vi "RealSense_HelloWorld_PointCloud_ext_RGB2.vi"() -> ()   [LabVIEW 2017]
doc: "Simple Demo showing how to connect a RealSense Camera to stream COLOR and DEPTH from the stereo camera of a D4xx series camera."
uses:
  libRealSense3.lvlib
  <vilib>/picture/3D Picture Control/NI_3D Picture Control.lvlib
  <vilib>/Utility/miscctls.llb/LV3DPointTypeDef.ctl
  <vilib>/Utility/miscctls.llb/LVRGBAColorTypeDef.ctl
  <vilib>/picture/3D Picture Control/Object/Create Object (name).vi
panel:
  in  "stop and exit":bool
  in  "Display tab":T1(tab)=enum."Color + Depth"
  out "RGB height":i32=720
  out "RGB width":i32=1280
  in  "Select RGB Resolution":u16(ring)=30 items=["320 x 180 @6fps", "320 x 180 @15fps", "320 x 180 @30fps", "320 x 180 @60fps", "320 x 240 @6fps", "320 x 240 @15fps", "320 x 240 @30fps", "320 x 240 @60fps", "424 x 240 @6fps", "424 x 240 @15fps", "424 x 240 @30fps", "424 x 240 @60fps", "640 x 360 @6fps", "640 x 360 @15fps", "640 x 360 @30fps", "640 x 360 @60fps", "640 x 480 @6fps", "640 x 480 @15fps", "640 x 480 @30fps", "640 x 480 @60fps", "848 x 480 @6fps", "848 x 480 @15fps", "848 x 480 @30fps", "848 x 480 @60fps", "960 x 540 @6fps", "960 x 540 @15fps", "960 x 540 @30fps", "960 x 540 @60fps", "1280 x 720 @6fps", "1280 x 720 @15fps", "1280 x 720 @30fps", "1920 x 1080 @6fps", "1920 x 1080 @15fps", "1920 x 1080 @30fps"]
  out "Depth height":i32=720
  out "Depth width":i32=1280
  out "init results":T2={"camera name"="Intel RealSense D435I", "camera S/N"="834412070342", "F/W"="05.12.01.00", "Sensor name"="Stereo Module", "api_version"=23201, "rscontext"=1659248689968, "device_list"=1659375430384, "device count"=1, "Dev out"=1659375543056, "sensor_list"=1659375327152, "sensor count"=3, "Sensor out"=1659374593968}
  in  "Select Depth Resolution":u16(ring)=32 items=["424 x 240 @6fps", "424 x 240 @15fps", "424 x 240 @30fps", "424 x 240 @60fps", "424 x 240 @90fps", "480 x 270 @6fps", "480 x 270 @15fps", "480 x 270 @30fps", "480 x 270 @60fps", "480 x 270 @90fps", "640 x 360 @6fps", "640 x 360 @15fps", "640 x 360 @30fps", "640 x 360 @60fps", "640 x 360 @90fps", "640 x 480 @6fps", "640 x 480 @15fps", "640 x 480 @30fps", "640 x 480 @60fps", "640 x 480 @90fps", "848 x 100 @6fps", "848 x 100 @15fps", "848 x 100 @30fps", "848 x 100 @60fps", "848 x 100 @90fps", "848 x 480 @6fps", "848 x 480 @15fps", "848 x 480 @30fps", "848 x 480 @60fps", "848 x 480 @90fps", "1280 x 720 @6fps", "1280 x 720 @15fps", "1280 x 720 @30fps", "1280 x 720 @60fps"]
  in  "Sensor index":i32
  in  "Device index":i32
  out "L-R Baseline, mm":sgl=-49.906834
  out "fy":sgl=656.61536 format="%#_5g"
  out "fx":sgl=656.61536 format="%#_5g"
  out "ppy":sgl=357.01468 format="%#_5g"
  out "ppx":sgl=632.28015 format="%#_5g"
  out "RGB Sensor":T3={"Sensor info"="RGB Camera", "Sensor out"=1659374594288, "error"=0}
  out "Stream Profile Handles":u64[](array[numeric])=[1659375449352]
  out "queue out":u64=1659245873280
  out "sensor out":u64=1659374594288
  out "Sensor out":u64=1659374594288
  out "Stream type":u16(ring)=2 items=["Depth"=0, "Color (ext.)"=2, "Color (left) "=3, "IR Left"=5, "IR Right"=9, "IR Left (Y16)"=21, "IR Right (Y16)"=25]
  in  "Exposure,us":sgl=33000.0
  in  "Autoexposure":bool=TRUE
  in  "Depth Presets":T4(ring)=enum."Face2"
  in  "Color Presets":T5(ring)=enum."DS410 (DS5a) 4"
  in  "Laser on/off":bool=TRUE
  in  "Gain(16-248)":sgl=16.0 min=16 max=248
  in  "Update Presets":bool
  in  "Laser \nPower (mW)":dbl(slide)=155.72448 min=0.0 max=360.0 scale=0.36..360.0
  in  "Range Scale":enum16{"200m", "100m", "60m", "6m", "2m", "1m"}(ring)=enum."6m"
  out "RGB image":picture
  out "Depth map":sgl[][](graph)
  out "3D Picture":refnum<vi>(3d-picture)
  out "RGB capture error":string="No Error"
  out "init error":string="\rNo Error\rNo Error\rNo Error\rNo Error\rNo Error\rNo Error\rNo Error\r\rNo Error\rNo Error"
  out "Depth Capture":string="No Error"
  out "Start Error":string="No Error\rNo Error\rNo Error"
  out "Config error":string="No Error\rNo Error"
  out "Close Error":string="No Error\rNo Error\rNo Error\rNo Error"
  out "release frame error":string="No Error"
  out "iteration":i32=762
  in  "stop":bool=TRUE
  # "RealSense Hello World: PointCloud ext. RGB"
  # "This demo shows how to connect a RealSense D435(e) & D415(e) Stereo Depth Camera, and display the textured PointCloud."
  # "Note; When you change Depth Preset you need to stop and restart for the HDAD settings to take effect.\n\nTry the Color preset called \"Remove IR2\". It will remove the laser projector from the RGB 1280x720 image."
  # "INTRINSICS & EXTRINSICS"
  # "SELECT THE RESOLUTION"
  # "DEPTH MAP"
  # "COLOR"
  # "Changes Color scale for Depth Map."
  # "20-1660000"
  # "3D POINTCLOUD"
  # "Rotate: Drag image\nMove X-Y: HOLD DOWN CTRL while dragging.\nZoom: SHIFT while dragging."
  # "ERRORS"
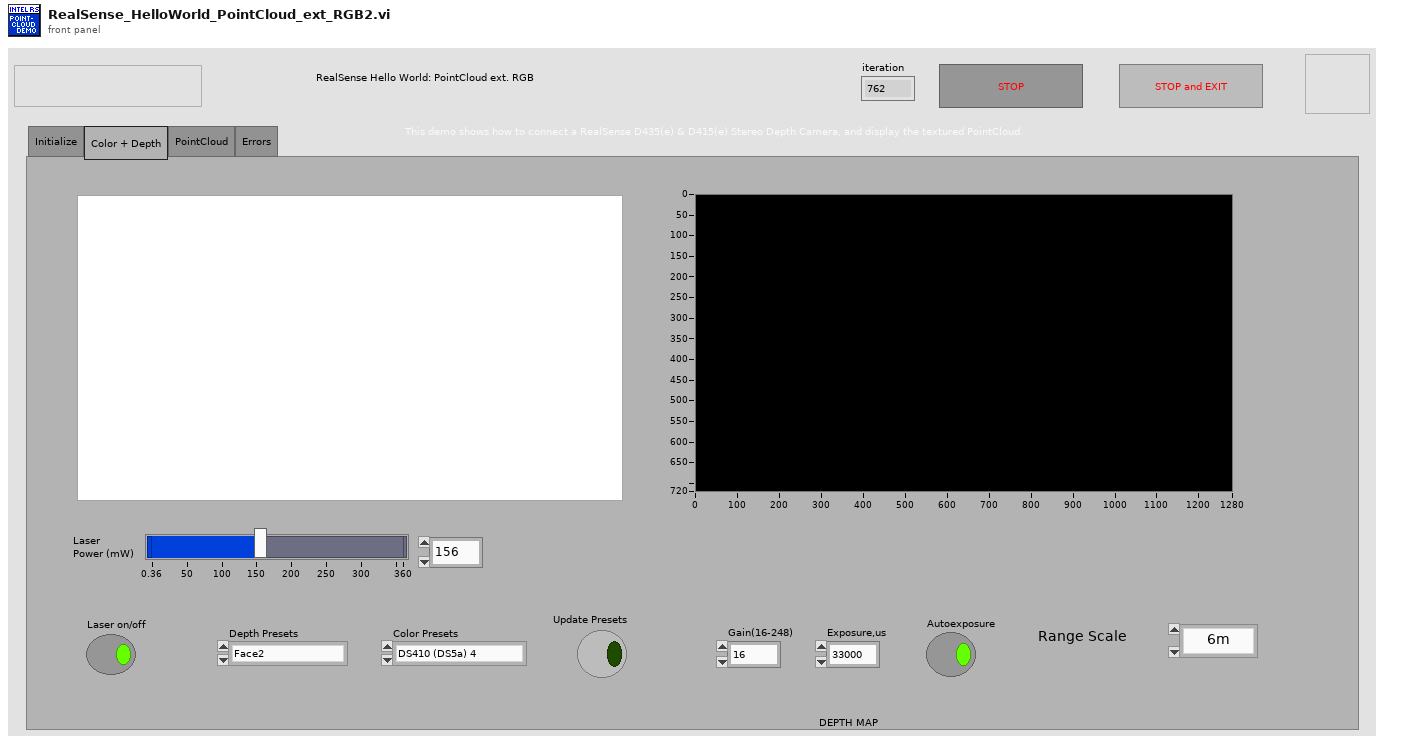
[diagram p1: front panel]
types:
  T1 = enum32{"Initialize", "Color + Depth", "PointCloud", "Errors"}
  T2 = cluster{"camera name":string, "camera S/N":string, "F/W":string, "Sensor name":string, "api_version":i32, "rscontext":u64, "device_list":u64, "device count":i32, "Dev out":u64, "sensor_list":u64, "sensor count":i32, "Sensor out":u64}
  T3 = cluster{"Sensor info":string, "Sensor out":u64, "error":u64}
  T4 = enum16{"Custom", "Original", "New Depth 1", "New Depth 2", "Depth Active 1", "Active 3D Scan", "Active Short A", "Active Short C", "Face", "Face2", "Best Box", "High Density", "Medium Density", "High Accuracy", "Hand", "Short Range", "Flat wall", "Load .JSON", "Load .JSON2"}
  T5 = enum16{"Custom", "RS400 (DS5p)", "RS400 (DS5p) 2", "RS400 (DS5p) 3", "RS400 (DS5p) 4", "RS400 (DS5p) 5", "RS410 (DS5a)", "RS410 (DS5a) 2", "DS410 (DS5a) 3", "DS410 (DS5a) 4", "DS410+IR", "DS5LR", "DS5LR-2", "DS5LR no pattern", "RS410 Remove IR", "RS410 Remove IR 2", "DS5micro", "D435"}
  T6 = cluster{"Sensor info":string, "Sensor out":u64, "error":u64}[]
  T7 = cluster{"width":i32, "height":i32, "fps":i32, "Profile":u64, "ppx":sgl, "ppy":sgl, "fx":sgl, "fy":sgl, "model":u32}
  T8 = enum16{"Overall", "Per Primitive", "Per Vertex", "Binding Off"}
  T9 = enum16{"Points", "Lines", "Line Strip", "Line Loop", "Triangles", "Triangle Strip", "Triangle Fan", "Quads", "Quad Strip", "Polygon"}
  T10 = cluster{"R":dbl, "G":dbl, "B":dbl, "Alpha":dbl}[]
  T11 = typedef "LVRGBAColorTypeDef.ctl" = cluster{"Red":sgl, "Green":sgl, "Blue":sgl, "Alpha":sgl}
  T12 = typedef "LV3DPointTypeDef.ctl" = cluster{"X":sgl, "Y":sgl, "Z":sgl}
  T13 = cluster{"Alpha":sgl, "Blue":sgl, "Green":sgl, "Red":sgl}
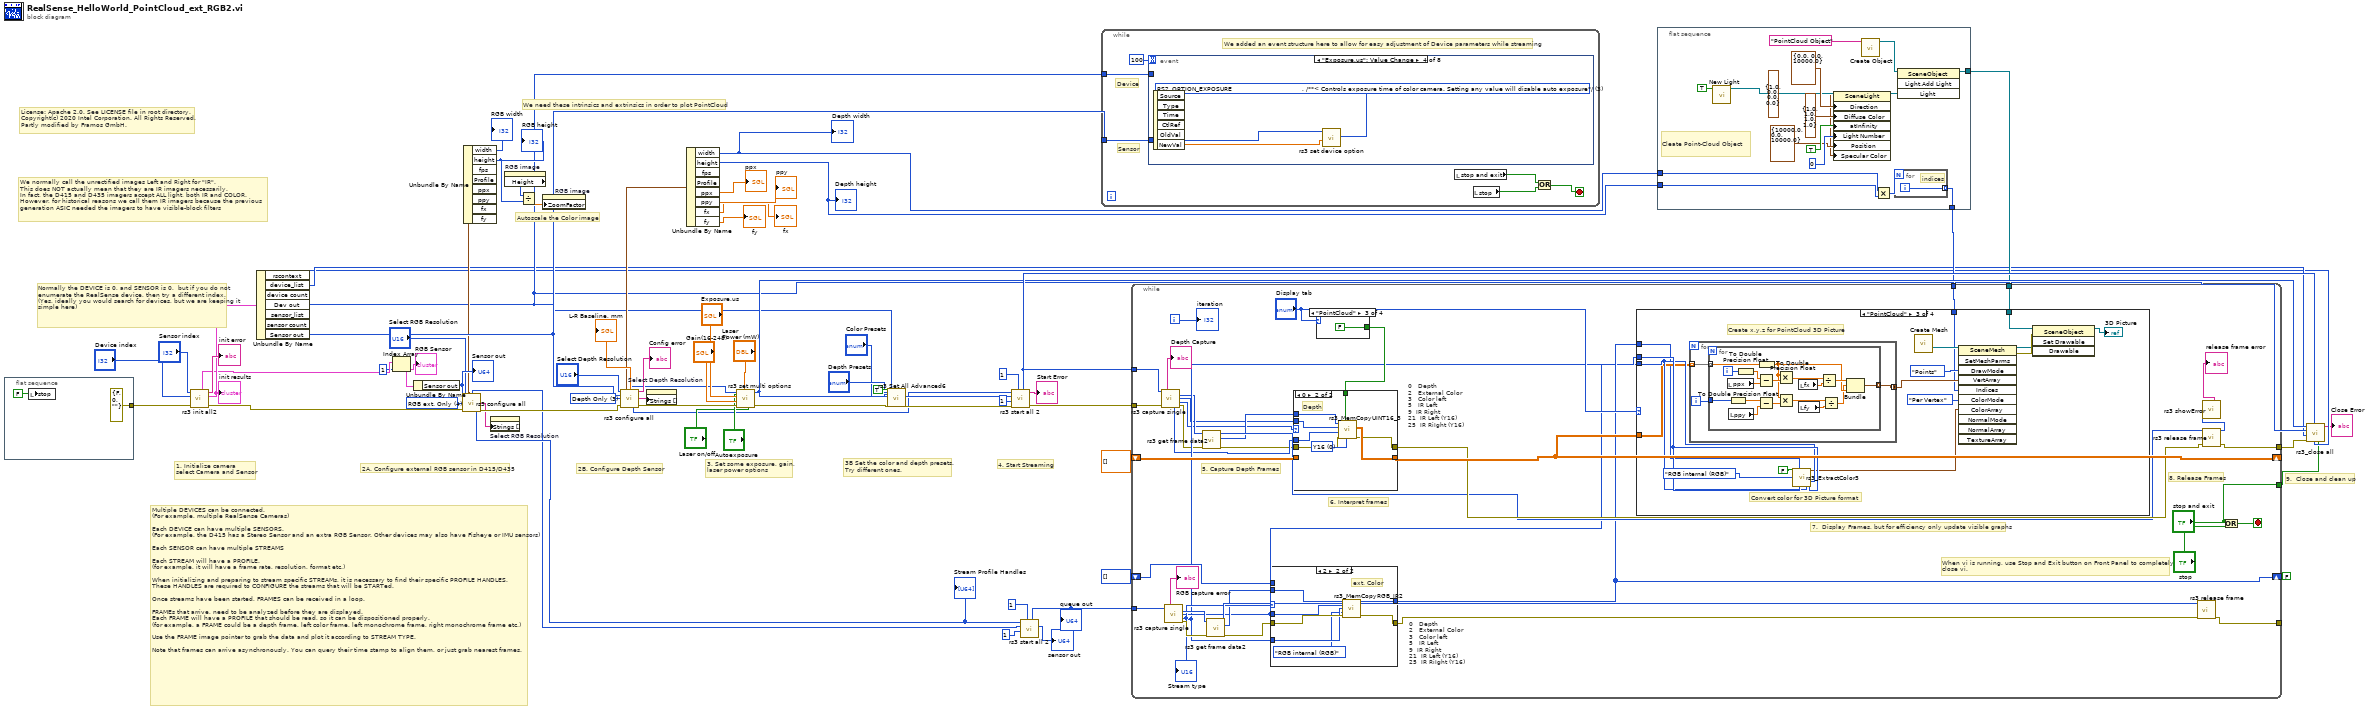
[diagram p0: block diagram]
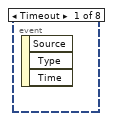
[diagram p2: hidden frame]
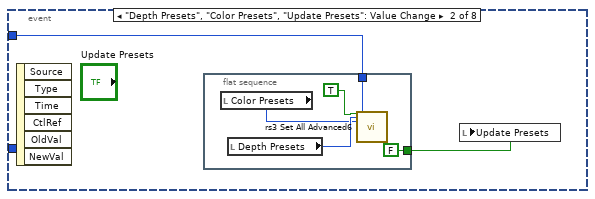
[diagram p3: hidden frame]
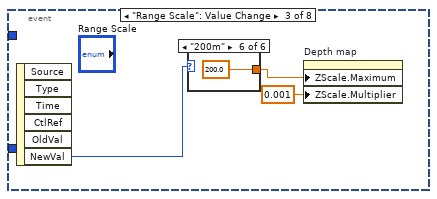
[diagram p4: hidden frame]
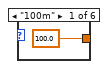
[diagram p5: hidden frame]
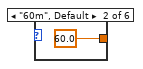
[diagram p6: hidden frame]
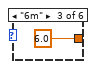
[diagram p7: hidden frame]
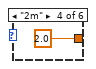
[diagram p8: hidden frame]
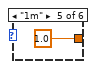
[diagram p9: hidden frame]
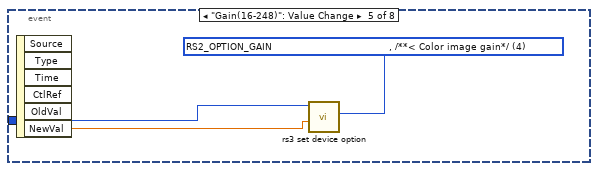
[diagram p10: hidden frame]
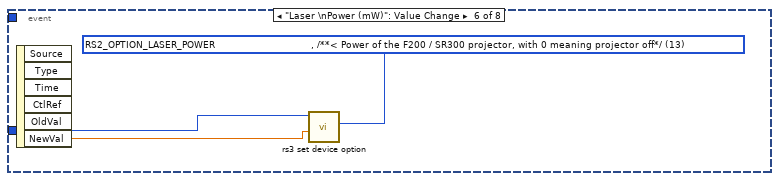
[diagram p11: hidden frame]
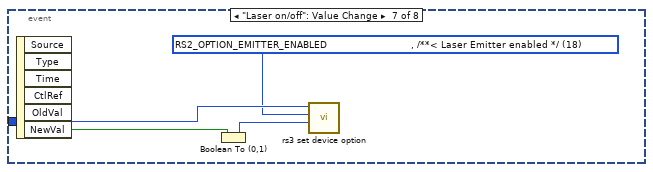
[diagram p12: hidden frame]
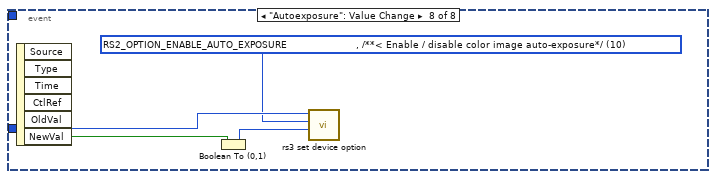
[diagram p13: hidden frame]
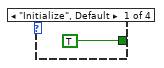
[diagram p16: hidden frame]
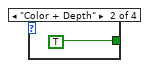
[diagram p17: hidden frame]
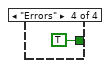
[diagram p18: hidden frame]
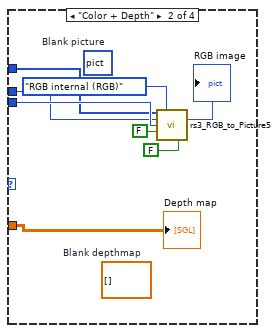
[diagram p20: hidden frame]
diagram:
  (unwired) FALSE
  w21 = u16 4 items=["Depth + Left Color", "Unrectified L + R", "Rectified L + R", "Depth Only", "RGB ext. Only"] ("Stream selection")
  w56 = u16 3 items=["Depth + Left Color", "Unrectified L + R", "Rectified L + R", "Depth Only", "RGB ext. Only"] ("Stream selection")
  # "License: Apache 2.0. See LICENSE file in root directory.\nCopyright(c) 2020 Intel Corporation. All Rights Reserved.\nPartly modified by Framos GmbH."
  # "2A. Configure external RGB sensor in D415/D435"
  # "Autoscale the Color image"
  # "We need these intrinsics and extrinsics in order to plot PointCloud"
  # "3B Set the color and depth presets.\nTry different ones."
  # "We normally call the unrectified images Left and Right for \"IR\". \nThis does NOT actually mean that they are IR imagers necessarily. \nIn fact, the D415 and D435 imagers accept ALL light, both IR and COLOR.\nHowever, for historical reasons we call them IR imagers because the previous generation ASIC needed the imagers to have visible-block filters"
  # "Normally the DEVICE is 0, and SENSOR is 0,  but if you do not enumerate the RealSense device, then try a different index.\n(Yes, ideally you would search for devices, but we are keeping it simple here)"
  # "Multiple DEVICES can be connected. \n(For example, multiple RealSense Cameras)\n\nEach DEVICE can have multiple SENSORS. \n(For example, the D415 has a Stereo Sensor and an extra RGB Sensor. Other devices may also have Fisheye or IMU sensors) \n\nEach SENSOR can have multiple STREAMS\n\nEach STREAM will have a PROFILE. \n(for example, it will have a frame rate, resolution, format etc.)\n\nWhen initializing and preparing to stream specific STREAMs, it is necessary to find their specific PROFILE HANDLES.\nThese HANDLES are required to CONFIGURE the streams that will be STARTed. \n\nOnce streams have been started, FRAMES can be received in a loop. \n \nFRAMEs that arrive, need to be analyzed before they are displayed. \nEach FRAME will have a PROFILE that should be read, so it can be dispositioned properly.\n(for example, a FRAME could be a depth frame, left color frame, left monochrome frame, right monochrome frame etc.)\n\nUse the FRAME image pointer to grab the data and plot it according to STREAM TYPE.\n\nNote that frames can arrive asynchronously. You can query their time stamp to align them, or just grab nearest frames."
  # "9.  Close and clean up"
  # "4. Start Streaming"
  # "3. Set some exposure, gain, \nlaser power options"
  # "2B. Configure Depth Sensor"
  # "1. Initialize camera\nselect Camera and Sensor"
  n1 = flat-sequence {
    tunnel: [errorcluster {"status"=FALSE, "code"=0, "source"=""} ("error in")] -> w57
    frame #0 {
      n2 = local write "stop"(FALSE ("stop")) -> ()
    }
  }
  n3 = call "rs3 init all2.vi"("error in"=w57, "Select Device"="Device index", "Select Sensor"="Sensor index") -> ("error out"=w27:errorcluster, "init results"=w62:T2, "init error"=→"init error":string, "Sensor Array"=w31:T6)  [unwired: 2 in, 3 out]
  "init results" <- w62
  n4 = Unbundle By Name(w62) -> ("rscontext"=w9:u64, "device_list"=w11:u64, "Dev out"=w12:u64, "Sensor out"=w44:u64)  [unwired: 3 out]
  n5 = Index Array(array=w31, index=1) -> (element=w29:T3)
  "RGB Sensor" <- w29
  n6 = Unbundle By Name(w29) -> ("Sensor out"=w28:u64)
  "Sensor out" <- w28
  n7 = call "rs3 configure all.vi"("Select Resolution"="Select RGB Resolution", "Sensor in"=w28, "Stream selection"=w21, "error in (no error)"=w27) -> ("Output stream L"=w24:T7, "Sensor out"=w18:u64, "Output stream"=w8:string[], "Stream Profile Handles"=w19:u64[], "error out"=w25:errorcluster)  [unwired: 2 in, 5 out]
  "Stream Profile Handles" <- w19
  n8 = Unbundle By Name(w24) -> ("width"=→"RGB width":i32, "height"=w22:i32)  [unwired: 6 out]
  "RGB height" <- w22
  n9 = property on="Select RGB Resolution" class="Ring (strict)"("Strings []"=w8) -> ()  [unwired: 2 in, 2 out]
  n10 = property on="RGB image" class="Pict"() -> ("Height"=w40:u32)  [unwired: 2 in, 2 out]
  n11 = Divide(x=w40, y=w22) -> (x/y=w39:dbl)
  n12 = property on="RGB image" class="Pict"("ZoomFactor"=w39) -> ()  [unwired: 2 in, 2 out]
  n13 = call "rs3 configure all.vi"("Select Resolution"="Select Depth Resolution", "Sensor in"=w44, "Stream selection"=w56, "error in (no error)"=w25) -> ("Output stream L"=w41:T7, "Sensor out"=w32:u64, "config error"=→"Config error":string, "Output stream"=w58:string[], "L-R Baseline, mm"=→"L-R Baseline, mm":sgl, "Stream Profile Handles"=w20:u64[], "error out"=w55:errorcluster)  [unwired: 2 in, 3 out]
  n14 = property on="Select Depth Resolution" class="Ring (strict)"("Strings []"=w58) -> ()  [unwired: 2 in, 2 out]
  n15 = Unbundle By Name(w41) -> ("width"=w3:i32, "height"=w2:i32, "ppx"=→"ppx":sgl, "ppy"=→"ppy":sgl, "fx"=→"fx":sgl, "fy"=→"fy":sgl)  [unwired: 2 out]
  "Depth height" <- w2
  "Depth width" <- w3
  n16 = call "rs3 set multi options.vi"("laser on/off"="Laser on/off", "autoexposure"="Autoexposure", "Laser power, mW (0-360)"="Laser \nPower (mW)", "error in (no error)"=w55, "Gain(16-248)"="Gain(16-248)", "Exposure, us"="Exposure,us", "Sensor in"=w32) -> ("error out"=w49:errorcluster, "Sensor out"=w54:u64)  [unwired: 2 in, 1 out]
  n17 = call "rs3 Set All Advanced6.vi"("Set Color Corr"=TRUE, "Depth Presets"="Depth Presets", "Color Presets"="Color Presets", "error in (no error)"=w49, "device in"=w12) -> ("error out"=w48:errorcluster)  [unwired: 20 in, 2 out]
  n18 = call "rs3 start all 2.vi"("capacity"=1, "error in (no error)"=w48, "Count of Streams"=1, "Sensor in"=w54, "Stream profile array"=w20) -> ("error out"=w59:errorcluster, "Config Error"=→"Start Error":string, "queue out"=w65:u64)  [unwired: 3 in, 1 out]
  n19 = call "rs3 start all 2.vi"("capacity"=1, "Count of Streams"=1, "Sensor in"=w18, "Stream profile array"=w19) -> ("sensor out"=→"sensor out":u64, "queue out"=w10:u64)  [unwired: 4 in, 2 out]
  "queue out" <- w10
  n20 = while {
    tunnel: w12 -> [w75]
    tunnel: w44 -> [w74]
    stop <- w70 stop-if-true
    # "Sensor"
    # "Device"
    # "We added an event structure here to allow for easy adjustment of Device parameters while streaming"
    n21 = event shown="[3] \"Exposure,us\": Value Change" {
      selector: _ -> [_ _ _ _ _ _ _ _]
      dyn-events: _ -> [_ _ _ _ _ _ _ _]
      timeout: 100 -> [_ _ _ _ _ _ _ _]
      tunnel: w75 -> [_ w77 _ _ _ _ _ _]
      tunnel: w74 -> [_ _ _ w94 w97 w100 w104 w108]
      event Timeout {
        n22 = event-data() -> ()  [unwired: 1 in, 3 out]
      }
      event "Depth Presets", "Color Presets", "Update Presets": Value Change {
        n23 = event-data() -> ()  [unwired: 1 in, 6 out]
        n24 = flat-sequence {
          tunnel: w77 -> [w79]
          tunnel: [FALSE ("Update Presets")] -> w76
          frame #0 {
            n25 = local read "Color Presets"() -> (w81:T5)
            n26 = local read "Depth Presets"() -> (w82:T4)
            n27 = call "rs3 Set All Advanced6.vi"("Set Color Corr"=TRUE, "Depth Presets"=w82, "Color Presets"=w81, "device in"=w79) -> ()  [unwired: 21 in, 3 out]
          }
        }
        n28 = local write "Update Presets"(w76) -> ()
      }
      event "Range Scale": Value Change {
        n29 = event-data() -> ("NewVal"=w84:enum16{"200m", "100m", "60m", "6m", "2m", "1m"})  [unwired: 1 in, 5 out]
        n30 = case shown="\"200m\"" w84 {
          tunnel: [100.0 ("Z Scale.Offset and Multiplier:Multiplier") 60.0 ("Z Scale.Offset and Multiplier:Multiplier") 6.0 ("Z Scale.Offset and Multiplier:Multiplier") 2.0 ("Z Scale.Offset and Multiplier:Multiplier") 1.0 ("Z Scale.Offset and Multiplier:Multiplier") 200.0 ("Z Scale.Offset and Multiplier:Multiplier")] -> w83
          frame "100m" {
          }
          frame "60m", Default {
          }
          frame "6m" {
          }
          frame "2m" {
          }
          frame "1m" {
          }
          frame "200m" {
          }
        }
        n31 = property on="Depth map" class="IntGraph (strict)"("ZScale.Maximum"=w83, "ZScale.Multiplier"=0.001 ("Z Scale.Offset and Multiplier:Multiplier")) -> ()  [unwired: 2 in, 2 out]
      }
      event "Exposure,us": Value Change {
        w92 = u16 3 items=["    RS2_OPTION_BACKLIGHT_COMPENSATION                     , /**< Enable / disable color backlight compensation*/", "    RS2_OPTION_BRIGHTNESS                                 , /**< Color image brightness*/", "    RS2_OPTION_CONTRAST                                   , /**< Color image contrast*/", "    RS2_OPTION_EXPOSURE                                   , /**< Controls exposure time of color camera. Setting any value will disable auto exposure*/", "    RS2_OPTION_GAIN                                       , /**< Color image gain*/", "    RS2_OPTION_GAMMA                                      , /**< Color image gamma setting*/", "    RS2_OPTION_HUE                                        , /**< Color image hue*/", "    RS2_OPTION_SATURATION                                 , /**< Color image saturation setting*/", "    RS2_OPTION_SHARPNESS                                  , /**< Color image sharpness setting*/", "    RS2_OPTION_WHITE_BALANCE                              , /**< Controls white balance of color image. Setting any value will disable auto white balance*/", "    RS2_OPTION_ENABLE_AUTO_EXPOSURE                       , /**< Enable / disable color image auto-exposure*/", "    RS2_OPTION_ENABLE_AUTO_WHITE_BALANCE                  , /**< Enable / disable color image auto-white-balance*/", "    RS2_OPTION_VISUAL_PRESET                              , /**< Provide access to several recommend sets of option presets for the depth camera */", "    RS2_OPTION_LASER_POWER                                , /**< Power of the F200 / SR300 projector, with 0 meaning projector off*/", "    RS2_OPTION_ACCURACY                                   , /**< Set the number of patterns projected per frame. The higher the accuracy value the more patterns projected. Increasing the number of patterns help to achieve better accuracy. Note that this c", "    RS2_OPTION_MOTION_RANGE                               , /**< Motion vs. Range trade-off, with lower values allowing for better motion sensitivity and higher values allowing for better depth range*/", "    RS2_OPTION_FILTER_OPTION                              , /**< Set the filter to apply to each depth frame. Each one of the filter is optimized per the application requirements*/", "    RS2_OPTION_CONFIDENCE_THRESHOLD                       , /**< The confidence level threshold used by the Depth algorithm pipe to set whether a pixel will get a valid range or will be marked with invalid range*/", "    RS2_OPTION_EMITTER_ENABLED                            , /**< Laser Emitter enabled */", "    RS2_OPTION_FRAMES_QUEUE_SIZE                          , /**< Number of frames the user is allowed to keep per stream. Trying to hold-on to more frames will cause frame-drops.*/", "    RS2_OPTION_TOTAL_FRAME_DROPS                          , /**< Total number of detected frame drops from all streams */", "    RS2_OPTION_AUTO_EXPOSURE_MODE                         , /**< Auto-Exposure modes: Static, Anti-Flicker and Hybrid */", "    RS2_OPTION_POWER_LINE_FREQUENCY                       , /**< Power Line Frequency control for anti-flickering Off/50Hz/60Hz/Auto */", "    RS2_OPTION_ASIC_TEMPERATURE                           , /**< Current Asic Temperature */", "    RS2_OPTION_ERROR_POLLING_ENABLED                      , /**< disable error handling */", "    RS2_OPTION_PROJECTOR_TEMPERATURE                      , /**< Current Projector Temperature */", "    RS2_OPTION_OUTPUT_TRIGGER_ENABLED                     , /**< Enable / disable trigger to be outputed from the camera to any external device on every depth frame */", "    RS2_OPTION_MOTION_MODULE_TEMPERATURE                  , /**< Current Motion-Module Temperature */", "    RS2_OPTION_DEPTH_UNITS                                , /**< Number of meters represented by a single depth unit */", "    RS2_OPTION_ENABLE_MOTION_CORRECTION                   , /**< Enable/Disable automatic correction of the motion data */", "    RS2_OPTION_AUTO_EXPOSURE_PRIORITY                     , /**< Allows sensor to dynamically ajust the frame rate depending on lighting conditions */", "    RS2_OPTION_COUNT                                      , /**< Number of enumeration values. Not a valid input: intended to be used in for-loops. */"] ("RS Option")
        n32 = event-data() -> ("NewVal"=w93:sgl)  [unwired: 1 in, 5 out]
        n33 = call "rs3 set device option.vi"("value"=w93, "RS Option"=w92, "Sensor in"=w94) -> ()  [unwired: 6 in, 3 out]
      }
      event "Gain(16-248)": Value Change {
        w95 = u16 4 items=["    RS2_OPTION_BACKLIGHT_COMPENSATION                     , /**< Enable / disable color backlight compensation*/", "    RS2_OPTION_BRIGHTNESS                                 , /**< Color image brightness*/", "    RS2_OPTION_CONTRAST                                   , /**< Color image contrast*/", "    RS2_OPTION_EXPOSURE                                   , /**< Controls exposure time of color camera. Setting any value will disable auto exposure*/", "    RS2_OPTION_GAIN                                       , /**< Color image gain*/", "    RS2_OPTION_GAMMA                                      , /**< Color image gamma setting*/", "    RS2_OPTION_HUE                                        , /**< Color image hue*/", "    RS2_OPTION_SATURATION                                 , /**< Color image saturation setting*/", "    RS2_OPTION_SHARPNESS                                  , /**< Color image sharpness setting*/", "    RS2_OPTION_WHITE_BALANCE                              , /**< Controls white balance of color image. Setting any value will disable auto white balance*/", "    RS2_OPTION_ENABLE_AUTO_EXPOSURE                       , /**< Enable / disable color image auto-exposure*/", "    RS2_OPTION_ENABLE_AUTO_WHITE_BALANCE                  , /**< Enable / disable color image auto-white-balance*/", "    RS2_OPTION_VISUAL_PRESET                              , /**< Provide access to several recommend sets of option presets for the depth camera */", "    RS2_OPTION_LASER_POWER                                , /**< Power of the F200 / SR300 projector, with 0 meaning projector off*/", "    RS2_OPTION_ACCURACY                                   , /**< Set the number of patterns projected per frame. The higher the accuracy value the more patterns projected. Increasing the number of patterns help to achieve better accuracy. Note that this c", "    RS2_OPTION_MOTION_RANGE                               , /**< Motion vs. Range trade-off, with lower values allowing for better motion sensitivity and higher values allowing for better depth range*/", "    RS2_OPTION_FILTER_OPTION                              , /**< Set the filter to apply to each depth frame. Each one of the filter is optimized per the application requirements*/", "    RS2_OPTION_CONFIDENCE_THRESHOLD                       , /**< The confidence level threshold used by the Depth algorithm pipe to set whether a pixel will get a valid range or will be marked with invalid range*/", "    RS2_OPTION_EMITTER_ENABLED                            , /**< Laser Emitter enabled */", "    RS2_OPTION_FRAMES_QUEUE_SIZE                          , /**< Number of frames the user is allowed to keep per stream. Trying to hold-on to more frames will cause frame-drops.*/", "    RS2_OPTION_TOTAL_FRAME_DROPS                          , /**< Total number of detected frame drops from all streams */", "    RS2_OPTION_AUTO_EXPOSURE_MODE                         , /**< Auto-Exposure modes: Static, Anti-Flicker and Hybrid */", "    RS2_OPTION_POWER_LINE_FREQUENCY                       , /**< Power Line Frequency control for anti-flickering Off/50Hz/60Hz/Auto */", "    RS2_OPTION_ASIC_TEMPERATURE                           , /**< Current Asic Temperature */", "    RS2_OPTION_ERROR_POLLING_ENABLED                      , /**< disable error handling */", "    RS2_OPTION_PROJECTOR_TEMPERATURE                      , /**< Current Projector Temperature */", "    RS2_OPTION_OUTPUT_TRIGGER_ENABLED                     , /**< Enable / disable trigger to be outputed from the camera to any external device on every depth frame */", "    RS2_OPTION_MOTION_MODULE_TEMPERATURE                  , /**< Current Motion-Module Temperature */", "    RS2_OPTION_DEPTH_UNITS                                , /**< Number of meters represented by a single depth unit */", "    RS2_OPTION_ENABLE_MOTION_CORRECTION                   , /**< Enable/Disable automatic correction of the motion data */", "    RS2_OPTION_AUTO_EXPOSURE_PRIORITY                     , /**< Allows sensor to dynamically ajust the frame rate depending on lighting conditions */", "    RS2_OPTION_COUNT                                      , /**< Number of enumeration values. Not a valid input: intended to be used in for-loops. */"] ("RS Option")
        n34 = event-data() -> ("NewVal"=w96:sgl)  [unwired: 1 in, 5 out]
        n35 = call "rs3 set device option.vi"("value"=w96, "RS Option"=w95, "Sensor in"=w97) -> ()  [unwired: 6 in, 3 out]
      }
      event "Laser \nPower (mW)": Value Change {
        w98 = u16 13 items=["    RS2_OPTION_BACKLIGHT_COMPENSATION                     , /**< Enable / disable color backlight compensation*/", "    RS2_OPTION_BRIGHTNESS                                 , /**< Color image brightness*/", "    RS2_OPTION_CONTRAST                                   , /**< Color image contrast*/", "    RS2_OPTION_EXPOSURE                                   , /**< Controls exposure time of color camera. Setting any value will disable auto exposure*/", "    RS2_OPTION_GAIN                                       , /**< Color image gain*/", "    RS2_OPTION_GAMMA                                      , /**< Color image gamma setting*/", "    RS2_OPTION_HUE                                        , /**< Color image hue*/", "    RS2_OPTION_SATURATION                                 , /**< Color image saturation setting*/", "    RS2_OPTION_SHARPNESS                                  , /**< Color image sharpness setting*/", "    RS2_OPTION_WHITE_BALANCE                              , /**< Controls white balance of color image. Setting any value will disable auto white balance*/", "    RS2_OPTION_ENABLE_AUTO_EXPOSURE                       , /**< Enable / disable color image auto-exposure*/", "    RS2_OPTION_ENABLE_AUTO_WHITE_BALANCE                  , /**< Enable / disable color image auto-white-balance*/", "    RS2_OPTION_VISUAL_PRESET                              , /**< Provide access to several recommend sets of option presets for the depth camera */", "    RS2_OPTION_LASER_POWER                                , /**< Power of the F200 / SR300 projector, with 0 meaning projector off*/", "    RS2_OPTION_ACCURACY                                   , /**< Set the number of patterns projected per frame. The higher the accuracy value the more patterns projected. Increasing the number of patterns help to achieve better accuracy. Note that this c", "    RS2_OPTION_MOTION_RANGE                               , /**< Motion vs. Range trade-off, with lower values allowing for better motion sensitivity and higher values allowing for better depth range*/", "    RS2_OPTION_FILTER_OPTION                              , /**< Set the filter to apply to each depth frame. Each one of the filter is optimized per the application requirements*/", "    RS2_OPTION_CONFIDENCE_THRESHOLD                       , /**< The confidence level threshold used by the Depth algorithm pipe to set whether a pixel will get a valid range or will be marked with invalid range*/", "    RS2_OPTION_EMITTER_ENABLED                            , /**< Laser Emitter enabled */", "    RS2_OPTION_FRAMES_QUEUE_SIZE                          , /**< Number of frames the user is allowed to keep per stream. Trying to hold-on to more frames will cause frame-drops.*/", "    RS2_OPTION_TOTAL_FRAME_DROPS                          , /**< Total number of detected frame drops from all streams */", "    RS2_OPTION_AUTO_EXPOSURE_MODE                         , /**< Auto-Exposure modes: Static, Anti-Flicker and Hybrid */", "    RS2_OPTION_POWER_LINE_FREQUENCY                       , /**< Power Line Frequency control for anti-flickering Off/50Hz/60Hz/Auto */", "    RS2_OPTION_ASIC_TEMPERATURE                           , /**< Current Asic Temperature */", "    RS2_OPTION_ERROR_POLLING_ENABLED                      , /**< disable error handling */", "    RS2_OPTION_PROJECTOR_TEMPERATURE                      , /**< Current Projector Temperature */", "    RS2_OPTION_OUTPUT_TRIGGER_ENABLED                     , /**< Enable / disable trigger to be outputed from the camera to any external device on every depth frame */", "    RS2_OPTION_MOTION_MODULE_TEMPERATURE                  , /**< Current Motion-Module Temperature */", "    RS2_OPTION_DEPTH_UNITS                                , /**< Number of meters represented by a single depth unit */", "    RS2_OPTION_ENABLE_MOTION_CORRECTION                   , /**< Enable/Disable automatic correction of the motion data */", "    RS2_OPTION_AUTO_EXPOSURE_PRIORITY                     , /**< Allows sensor to dynamically ajust the frame rate depending on lighting conditions */", "    RS2_OPTION_COUNT                                      , /**< Number of enumeration values. Not a valid input: intended to be used in for-loops. */"] ("RS Option")
        n36 = event-data() -> ("NewVal"=w99:dbl)  [unwired: 1 in, 5 out]
        n37 = call "rs3 set device option.vi"("value"=w99, "RS Option"=w98, "Sensor in"=w100) -> ()  [unwired: 6 in, 3 out]
      }
      event "Laser on/off": Value Change {
        w103 = u16 18 items=["    RS2_OPTION_BACKLIGHT_COMPENSATION                     , /**< Enable / disable color backlight compensation*/", "    RS2_OPTION_BRIGHTNESS                                 , /**< Color image brightness*/", "    RS2_OPTION_CONTRAST                                   , /**< Color image contrast*/", "    RS2_OPTION_EXPOSURE                                   , /**< Controls exposure time of color camera. Setting any value will disable auto exposure*/", "    RS2_OPTION_GAIN                                       , /**< Color image gain*/", "    RS2_OPTION_GAMMA                                      , /**< Color image gamma setting*/", "    RS2_OPTION_HUE                                        , /**< Color image hue*/", "    RS2_OPTION_SATURATION                                 , /**< Color image saturation setting*/", "    RS2_OPTION_SHARPNESS                                  , /**< Color image sharpness setting*/", "    RS2_OPTION_WHITE_BALANCE                              , /**< Controls white balance of color image. Setting any value will disable auto white balance*/", "    RS2_OPTION_ENABLE_AUTO_EXPOSURE                       , /**< Enable / disable color image auto-exposure*/", "    RS2_OPTION_ENABLE_AUTO_WHITE_BALANCE                  , /**< Enable / disable color image auto-white-balance*/", "    RS2_OPTION_VISUAL_PRESET                              , /**< Provide access to several recommend sets of option presets for the depth camera */", "    RS2_OPTION_LASER_POWER                                , /**< Power of the F200 / SR300 projector, with 0 meaning projector off*/", "    RS2_OPTION_ACCURACY                                   , /**< Set the number of patterns projected per frame. The higher the accuracy value the more patterns projected. Increasing the number of patterns help to achieve better accuracy. Note that this c", "    RS2_OPTION_MOTION_RANGE                               , /**< Motion vs. Range trade-off, with lower values allowing for better motion sensitivity and higher values allowing for better depth range*/", "    RS2_OPTION_FILTER_OPTION                              , /**< Set the filter to apply to each depth frame. Each one of the filter is optimized per the application requirements*/", "    RS2_OPTION_CONFIDENCE_THRESHOLD                       , /**< The confidence level threshold used by the Depth algorithm pipe to set whether a pixel will get a valid range or will be marked with invalid range*/", "    RS2_OPTION_EMITTER_ENABLED                            , /**< Laser Emitter enabled */", "    RS2_OPTION_FRAMES_QUEUE_SIZE                          , /**< Number of frames the user is allowed to keep per stream. Trying to hold-on to more frames will cause frame-drops.*/", "    RS2_OPTION_TOTAL_FRAME_DROPS                          , /**< Total number of detected frame drops from all streams */", "    RS2_OPTION_AUTO_EXPOSURE_MODE                         , /**< Auto-Exposure modes: Static, Anti-Flicker and Hybrid */", "    RS2_OPTION_POWER_LINE_FREQUENCY                       , /**< Power Line Frequency control for anti-flickering Off/50Hz/60Hz/Auto */", "    RS2_OPTION_ASIC_TEMPERATURE                           , /**< Current Asic Temperature */", "    RS2_OPTION_ERROR_POLLING_ENABLED                      , /**< disable error handling */", "    RS2_OPTION_PROJECTOR_TEMPERATURE                      , /**< Current Projector Temperature */", "    RS2_OPTION_OUTPUT_TRIGGER_ENABLED                     , /**< Enable / disable trigger to be outputed from the camera to any external device on every depth frame */", "    RS2_OPTION_MOTION_MODULE_TEMPERATURE                  , /**< Current Motion-Module Temperature */", "    RS2_OPTION_DEPTH_UNITS                                , /**< Number of meters represented by a single depth unit */", "    RS2_OPTION_ENABLE_MOTION_CORRECTION                   , /**< Enable/Disable automatic correction of the motion data */", "    RS2_OPTION_AUTO_EXPOSURE_PRIORITY                     , /**< Allows sensor to dynamically ajust the frame rate depending on lighting conditions */", "    RS2_OPTION_COUNT                                      , /**< Number of enumeration values. Not a valid input: intended to be used in for-loops. */"] ("RS Option")
        n38 = event-data() -> ("NewVal"=w102:bool)  [unwired: 1 in, 5 out]
        n39 = Boolean To (0,1)(Boolean=w102) -> (0, 1=w101:i16)
        n40 = call "rs3 set device option.vi"("value"=w101, "RS Option"=w103, "Sensor in"=w104) -> ()  [unwired: 6 in, 3 out]
      }
      event "Autoexposure": Value Change {
        w107 = u16 10 items=["    RS2_OPTION_BACKLIGHT_COMPENSATION                     , /**< Enable / disable color backlight compensation*/", "    RS2_OPTION_BRIGHTNESS                                 , /**< Color image brightness*/", "    RS2_OPTION_CONTRAST                                   , /**< Color image contrast*/", "    RS2_OPTION_EXPOSURE                                   , /**< Controls exposure time of color camera. Setting any value will disable auto exposure*/", "    RS2_OPTION_GAIN                                       , /**< Color image gain*/", "    RS2_OPTION_GAMMA                                      , /**< Color image gamma setting*/", "    RS2_OPTION_HUE                                        , /**< Color image hue*/", "    RS2_OPTION_SATURATION                                 , /**< Color image saturation setting*/", "    RS2_OPTION_SHARPNESS                                  , /**< Color image sharpness setting*/", "    RS2_OPTION_WHITE_BALANCE                              , /**< Controls white balance of color image. Setting any value will disable auto white balance*/", "    RS2_OPTION_ENABLE_AUTO_EXPOSURE                       , /**< Enable / disable color image auto-exposure*/", "    RS2_OPTION_ENABLE_AUTO_WHITE_BALANCE                  , /**< Enable / disable color image auto-white-balance*/", "    RS2_OPTION_VISUAL_PRESET                              , /**< Provide access to several recommend sets of option presets for the depth camera */", "    RS2_OPTION_LASER_POWER                                , /**< Power of the F200 / SR300 projector, with 0 meaning projector off*/", "    RS2_OPTION_ACCURACY                                   , /**< Set the number of patterns projected per frame. The higher the accuracy value the more patterns projected. Increasing the number of patterns help to achieve better accuracy. Note that this c", "    RS2_OPTION_MOTION_RANGE                               , /**< Motion vs. Range trade-off, with lower values allowing for better motion sensitivity and higher values allowing for better depth range*/", "    RS2_OPTION_FILTER_OPTION                              , /**< Set the filter to apply to each depth frame. Each one of the filter is optimized per the application requirements*/", "    RS2_OPTION_CONFIDENCE_THRESHOLD                       , /**< The confidence level threshold used by the Depth algorithm pipe to set whether a pixel will get a valid range or will be marked with invalid range*/", "    RS2_OPTION_EMITTER_ENABLED                            , /**< Laser Emitter enabled */", "    RS2_OPTION_FRAMES_QUEUE_SIZE                          , /**< Number of frames the user is allowed to keep per stream. Trying to hold-on to more frames will cause frame-drops.*/", "    RS2_OPTION_TOTAL_FRAME_DROPS                          , /**< Total number of detected frame drops from all streams */", "    RS2_OPTION_AUTO_EXPOSURE_MODE                         , /**< Auto-Exposure modes: Static, Anti-Flicker and Hybrid */", "    RS2_OPTION_POWER_LINE_FREQUENCY                       , /**< Power Line Frequency control for anti-flickering Off/50Hz/60Hz/Auto */", "    RS2_OPTION_ASIC_TEMPERATURE                           , /**< Current Asic Temperature */", "    RS2_OPTION_ERROR_POLLING_ENABLED                      , /**< disable error handling */", "    RS2_OPTION_PROJECTOR_TEMPERATURE                      , /**< Current Projector Temperature */", "    RS2_OPTION_OUTPUT_TRIGGER_ENABLED                     , /**< Enable / disable trigger to be outputed from the camera to any external device on every depth frame */", "    RS2_OPTION_MOTION_MODULE_TEMPERATURE                  , /**< Current Motion-Module Temperature */", "    RS2_OPTION_DEPTH_UNITS                                , /**< Number of meters represented by a single depth unit */", "    RS2_OPTION_ENABLE_MOTION_CORRECTION                   , /**< Enable/Disable automatic correction of the motion data */", "    RS2_OPTION_AUTO_EXPOSURE_PRIORITY                     , /**< Allows sensor to dynamically ajust the frame rate depending on lighting conditions */", "    RS2_OPTION_COUNT                                      , /**< Number of enumeration values. Not a valid input: intended to be used in for-loops. */"] ("RS Option")
        n41 = event-data() -> ("NewVal"=w106:bool)  [unwired: 1 in, 5 out]
        n42 = Boolean To (0,1)(Boolean=w106) -> (0, 1=w105:i16)
        n43 = call "rs3 set device option.vi"("value"=w105, "RS Option"=w107, "Sensor in"=w108) -> ()  [unwired: 6 in, 3 out]
      }
    }
    n44 = local read "stop and exit"() -> (w71:bool)
    n45 = local read "stop"() -> (w72:bool)
    n46 = Or(x=w71, y=w72) -> (x .or. y?=w70:bool)
  }
  n47 = while {
    tunnel: w65 -> [w143]
    tunnel: w59 -> [w147]
    tunnel: [w145] -> w64
    shift-right: [w137] -> _
    shift-left: sgl[][] [] ("2D Array Output") -> [w142]
    tunnel: w34 -> [w141]
    tunnel: w33 -> [w140]
    tunnel: w10 -> [w134]
    tunnel: [w128] -> _
    shift-right: [w127] -> _
    shift-left: u8[] [] ("Output Array") -> [w125]
    tunnel: ["stop and exit"] -> w1
    i -> [w146]
    stop <- w111 stop-if-true
    # "When vi is running, use Stop and Exit button on Front Panel to completely\nclose vi."
    # "0   Depth\n2   External Color \n3   Color left\n5   IR Left \n9  IR Right\n21  IR Left (Y16)\n25  IR RiIght (Y16)"
    # "0   Depth\n2   External Color \n3   Color left\n5   IR Left \n9  IR Right\n21  IR Left (Y16)\n25  IR RiIght (Y16)"
    # "6. Interpret frames"
    # "5. Capture Depth Frames"
    # "8. Release Frames"
    # "7.  Display Frames, but for efficiency only update visible graphs"
    n48 = call "rs3 capture single.vi"("queue in"=w143, "error in (no error)"=w147) -> ("Capture Error"=→"Depth Capture":string, "frame out"=w120:u64, "width"=w117:i32, "Stream type"=w118:u16, "height"=w116:i32, "error out"=w114:errorcluster)  [unwired: 5 in, 3 out]
    n49 = call "rs3 capture single.vi"("queue in"=w134) -> ("Capture Error"=→"RGB capture error":string, "frame out"=w131:u64, "width"=w122:i32, "Stream type"=w124:u16, "height"=w121:i32, "error out"=w132:errorcluster)  [unwired: 6 in, 3 out]
    "Stream type" <- w124
    n50 = call "rs3 get frame data2.vi"("error in (no error)"=w114, "frame in"=w120) -> ("error out"=w115:errorcluster, "image pointer out"=w119:u64, "Frame out"=w135:u64)  [unwired: 6 in, 1 out]
    n51 = call "rs3 get frame data2.vi"("error in (no error)"=w132, "frame in"=w131) -> ("error out"=w130:errorcluster, "image pointer out"=w123:u64, "Frame out"=w126:u64)  [unwired: 6 in, 1 out]
    n52 = case shown="2" w124 {
      tunnel: [w159 w165] -> w129
      tunnel: w123 -> [_ w166]
      tunnel: w130 -> [w159 w164]
      tunnel: w122 -> [_ w163]
      tunnel: w121 -> [_ w162]
      tunnel: [w158 w161] -> w127
      tunnel: w125 -> [w158 _]
      frame 1, Default {
      }
      frame 2 {
        # "ext. Color"
        n53 = call "rs3_MemCopyRGB_IR2.vi"("Zimage pointer"=w166, "RGB  X, width"=w163, "RGB Y, height"=w162, "Color format"=enum16{"Monochrome", "RGB internal (RGB)"}."RGB internal (RGB)", "error in (no error)"=w164) -> ("Output Array"=w161:u8[], "error out"=w165:errorcluster)  [unwired: 8 in, 1 out]
      }
    }
    n54 = case shown="\"PointCloud\"" "Display tab" {
      tunnel: [TRUE ("Transpose") TRUE ("Transpose") FALSE ("Transpose") TRUE ("Transpose")] -> w138
      frame "Initialize", Default {
      }
      frame "Color + Depth" {
      }
      frame "PointCloud" {
      }
      frame "Errors" {
      }
    }
    n55 = case shown="0" w118 {
      tunnel: [w149 w154] -> w136
      tunnel: w119 -> [_ w153]
      tunnel: w117 -> [_ w152]
      tunnel: w116 -> [_ w151]
      tunnel: w115 -> [w149 w155]
      tunnel: [w148 w156] -> w137
      tunnel: w142 -> [w148 _]
      tunnel: w138 -> [_ w150]
      frame 1, Default {
      }
      frame 0 {
        w157 = u16 0 items=["Y16", "Y8"] ("Image format")
        # "Depth"
        n56 = call "rs3_MemCopyUINT16_3.vi"("Image format"=w157, "Transpose"=w150, "error in (no error)"=w155, "Depth Y"=w151, "Depth X"=w152, "Zimage pointer"=w153) -> ("error out"=w154:errorcluster, "2D Array Output"=w156:sgl[][])  [unwired: 2 in, 2 out]
      }
    }
    n57 = case shown="\"PointCloud\"" "Display tab" {
      tunnel: w122 -> [_ w172 w194 _]
      tunnel: w121 -> [_ w178 w193 _]
      tunnel: w137 -> [_ w177 w181 _]
      tunnel: w141 -> [_ _ w183 _]
      tunnel: w140 -> [_ _ w182 _]
      tunnel: w127 -> [_ w176 w180 _]
      frame "Initialize", Default {
      }
      frame "Color + Depth" {
        (unwired) picture bytes[33]  # Blank picture
        (unwired) sgl[][] []  # Blank depthmap
        n58 = call "rs3_RGB_to_Picture5.vi"("RGB array"=w176, "Color format"=enum16{"Monochrome", "RGB internal (RGB)"}."RGB internal (RGB)", "RGB  X, width"=w172, "RGB Y, height"=w178, "AWB"=FALSE, "White Balance"=FALSE) -> ("new picture"=→"RGB image":picture)  [unwired: 8 in, 1 out]
        "Depth map" <- w177
      }
      frame "PointCloud" {
        # "Convert color for 3D Picture format"
        # "Create x,y,z for PointCloud 3D Picture"
        n59 = for {
          tunnel: w181 -> [w197] mode=indexing
          tunnel: [w196] -> w187 mode=concatenating
          i -> [w195]
          n60 = for {
            tunnel: w197 -> [w214] mode=indexing
            tunnel: w195 -> [w213]
            tunnel: [w212] -> w196 mode=indexing
            i -> [w211]
            n61 = local read "ppx"() -> (w204:sgl)
            n62 = local read "ppy"() -> (w202:sgl)
            n63 = To Double Precision Float(number=w213) -> (double precision float=w201:dbl)
            n64 = To Double Precision Float(number=w211) -> (double precision float=w206:dbl)
            n65 = Subtract(x=w206, y=w204) -> (x-y=w205:dbl)
            n66 = Subtract(x=w201, y=w202) -> (x-y=w200:dbl)
            n67 = To Double Precision Float(number=w214) -> (double precision float=w199:dbl)
            n68 = Multiply(x=w199, y=w205) -> (x*y=w210:dbl)
            n69 = Multiply(x=w199, y=w200) -> (x*y=w207:dbl)
            n70 = local read "fx"() -> (w209:sgl)
            n71 = local read "fy"() -> (w203:sgl)
            n72 = Divide(x=w210, y=w209) -> (x/y=w208:dbl)
            n73 = Divide(x=w207, y=w203) -> (x/y=w198:dbl)
            n74 = Bundle(w208, w198, w199) -> (w212:cluster{dbl, dbl, dbl})  [unwired: 1 in]
          }
        }
        n75 = call "rs3_ExtractColor3.vi"("White Balance"=FALSE, "24bit Color Array"=w180, "Color format"=enum16{"Monochrome", "RGB internal (RGB)"}."RGB internal (RGB)", "Depth Y"=w193, "RGB  X"=w194, "RGB Y"=w193, "Depth X"=w194) -> ("Norm Mesh Color"=w186:T10)  [unwired: 8 in]
        n76 = call <vilib>:"Create Mesh.vi"() -> ("New Mesh Refnum"=w189:refnum<vi>)  [unwired: 10 in, 1 out]
        n77 = invoke class="SceneMesh" method="SetMeshParms"(reference=w189, "DrawMode"=T9."Points" ("Draw Mode"), "VertArray"=w187, "Indices"=w182, "ColorMode"=T8."Per Vertex" ("Color Binding Mode"), "ColorArray"=w186) -> (reference out=w190:refnum<vi>, error out=w191:errorcluster)  [unwired: 5 in, 9 out]
        n78 = invoke class="SceneObject" method="Set Drawable"(reference=w183, error in=w191, "Drawable"=w190) -> (reference out=→"3D Picture":refnum<vi>)  [unwired: 1 in, 3 out]
      }
      frame "Errors" {
      }
    }
    n79 = call "rs3 release frame.vi"("error in (no error)"=w129, "Frame"=w126) -> ("error out"=w128:errorcluster)  [unwired: 8 in, 1 out]
    n80 = call "rs3 release frame.vi"("error in (no error)"=w136, "Frame"=w135) -> ("error out"=w145:errorcluster, "error"=w112:u64)  [unwired: 8 in]
    n81 = call "rs3 showError.vi"("error"=w112) -> ("Error summary"=→"release frame error":string)  [unwired: 6 in, 4 out]
    n82 = Or(x="stop and exit", y="stop") -> (x .or. y?=w111:bool)
    "iteration" <- w146
  }
  n83 = flat-sequence {
    tunnel: [w219] -> w34
    tunnel: [w217] -> w33
    tunnel: w3 -> [w216]
    tunnel: w2 -> [w215]
    frame #0 {
      # "Cleate Point-Cloud Object"
      n84 = call <vilib>:"New Light.vi"("At Infinity"=TRUE) -> ("New Light Refnum"=w227:refnum<vi>)  [unwired: 2 in, 8 out]
      n85 = property class="SceneLight"(reference=w227, "Direction"=cluster{"X":sgl, "Y":sgl, "Z":sgl} {"X"=0.0, "Y"=0.0, "Z"=10000.0}, "Diffuse Color"=T13 {"Alpha"=1.0, "Blue"=1.0, "Green"=1.0, "Red"=1.0}, "atInfinity"=TRUE ("At Infinity"), "Light Number"=0, "Position"=T12 {"X"=10000.0, "Y"=0.0, "Z"=10000.0}, "Specular Color"=T11 {"Red"=1.0, "Green"=0.0, "Blue"=0.0, "Alpha"=0.0}) -> (reference out=w224:refnum<vi>)  [unwired: 1 in, 1 out]
      n86 = call-poly <vilib>:"Create Object.vi"("Name"="PointCloud Object") -> ("Scene:New Object"=w226:refnum<vi>)  [unwired: 9 in, 1 out]
      n87 = Multiply(x=w216, y=w215) -> (x*y=w218:i32)
      n88 = for {
        N: w218 -> [_]
        tunnel: [w231] -> w217 mode=indexing
        i -> [w231]
        # "indices"
      }
      n89 = invoke class="SceneObject" method="Light.Add Light"(reference=w226, "Light"=w224) -> (reference out=w219:refnum<vi>)  [unwired: 2 in, 3 out]
    }
  }
  n90 = call "rs3_close all.vi"("Stop and Exit"=w1, "rscontext"=w9, "queue in"=w65, "error in (no error)"=w64, "device_list"=w11, "Dev in"=w12, "Sensor in"=w54) -> ("Close Error"=→"Close Error":string)  [unwired: 3 in, 1 out]
